vi "ReadDAQTask.vi"(8 "Error In":errorcluster, 11 "DAQ Task In":refnum<k21>) -> (0 "Error Out":errorcluster, 2 "Data":dbl[][](array[numeric]), 3 "DAQ Task Out":refnum<k21>)   [LabVIEW 2012]
uses:
  <vilib>/DAQmx/read.llb/DAQmx Read (Analog 2D DBL NChan NSamp).vi
  <vilib>/DAQmx/miscellaneous.llb/DAQmx Fill In Error Info.vi
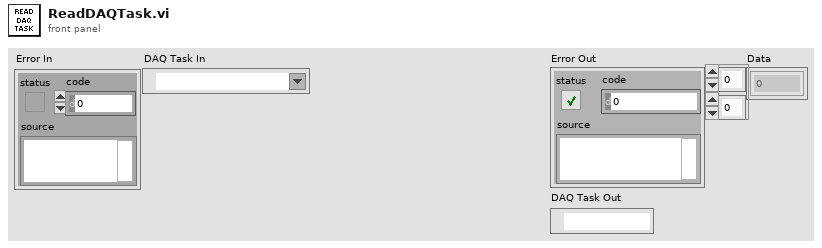
[diagram p1: front panel]
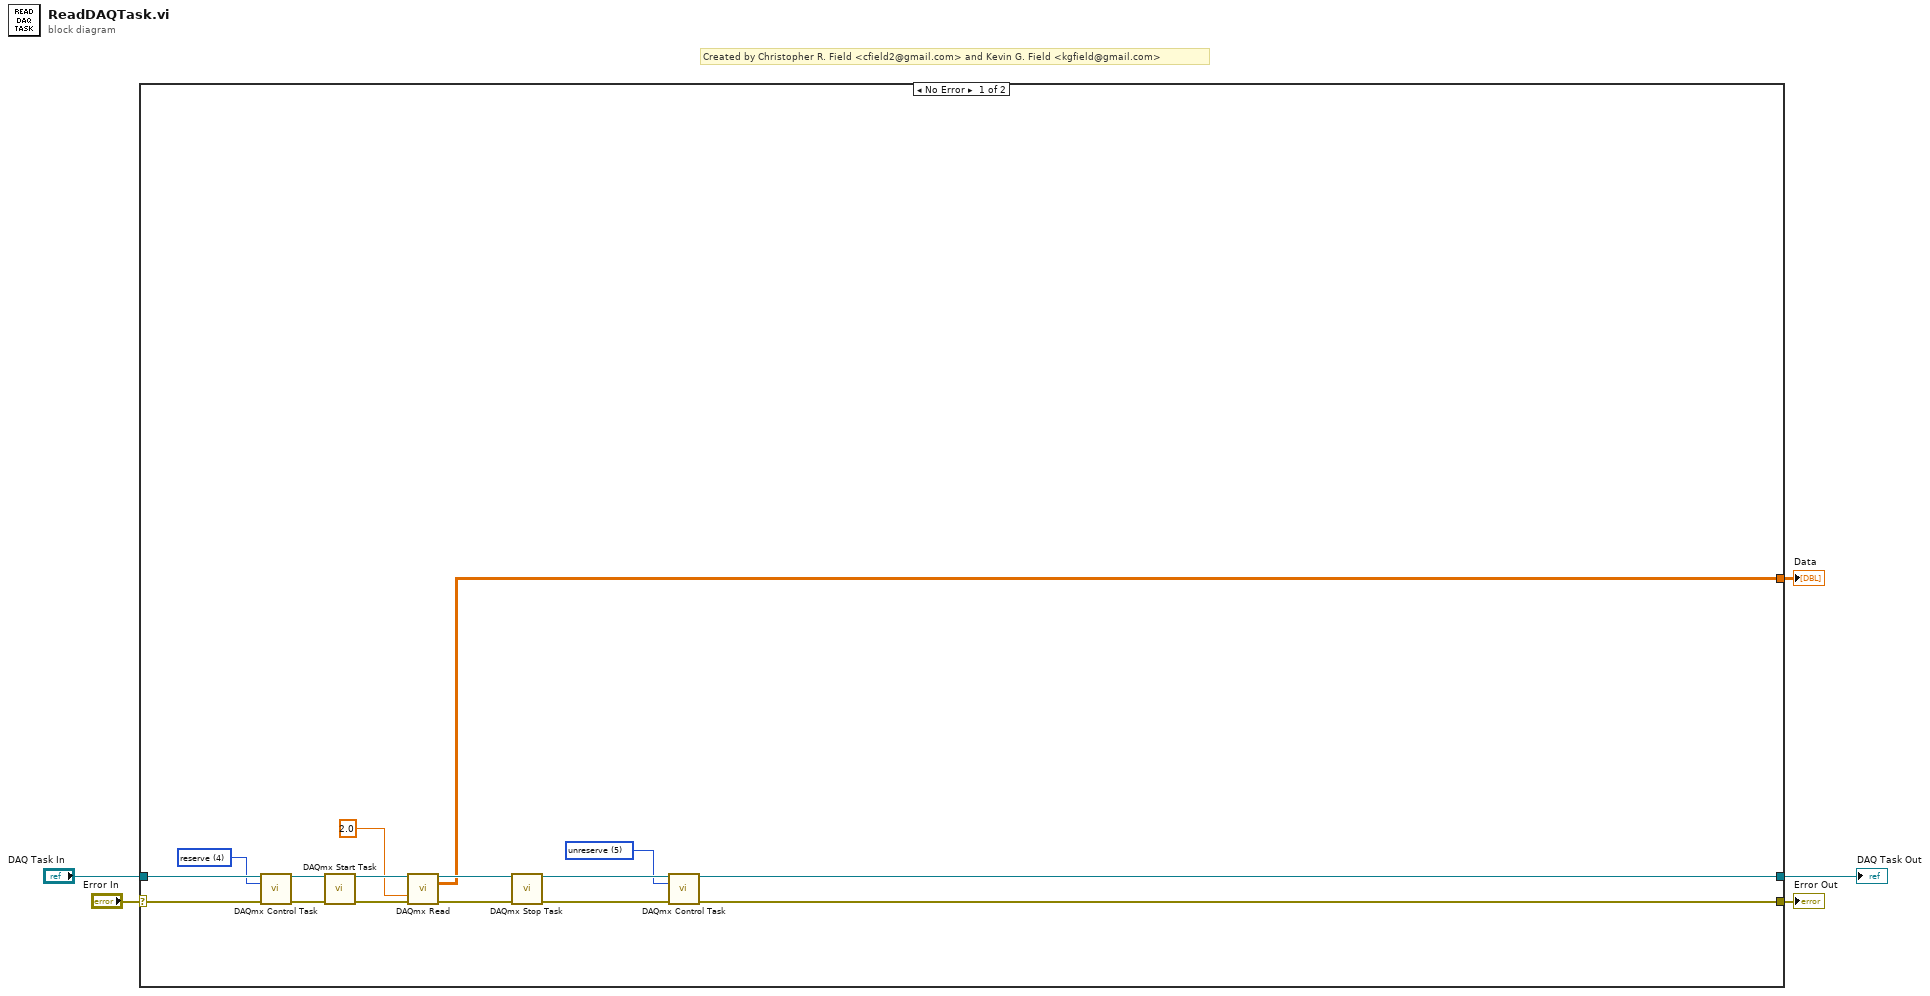
[diagram p0: block diagram]
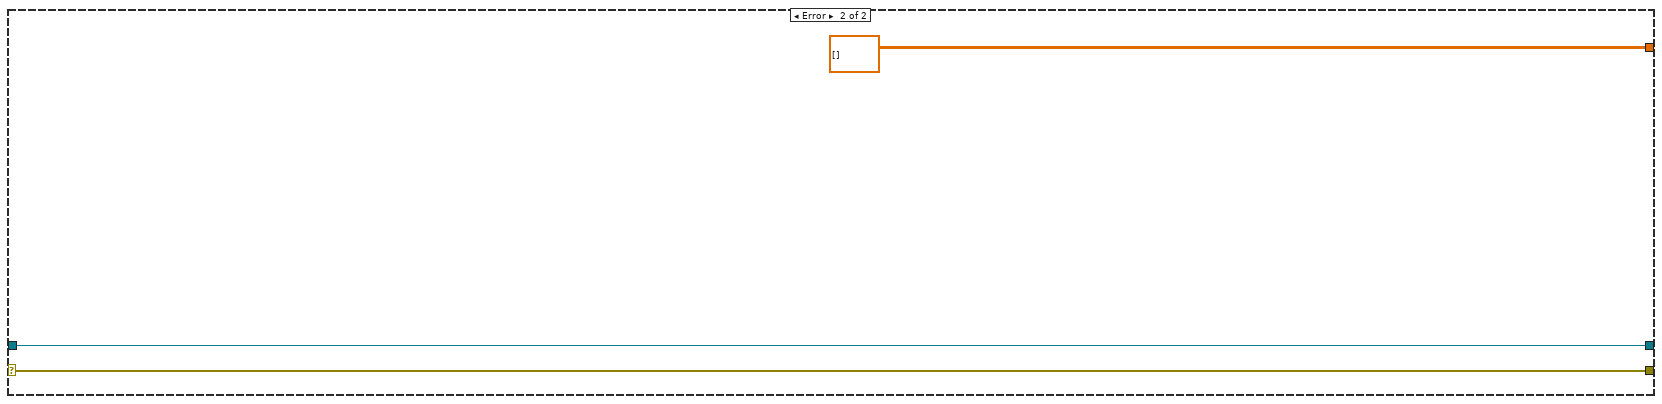
[diagram p2: hidden frame]
diagram:
  # "Created by Christopher R. Field <cfield2@gmail.com> and Kevin G. Field <kgfield@gmail.com>"
  n1 = case shown="No Error" "Error In" {
    selector: "Error In" -> [w11 w23]
    tunnel: [w8 w23] -> w4
    tunnel: "DAQ Task In" -> [w14 w24]
    tunnel: [w7 w24] -> w2
    tunnel: [w17 dbl[][] [] ("data")] -> w1
    frame No Error {
      w9 = 5 items=["verify"=2, "reserve"=4, "commit"=3, "unreserve"=5, "abort"=6] ("action")
      w10 = 4 items=["verify"=2, "reserve"=4, "commit"=3, "unreserve"=5, "abort"=6] ("action")
      n2 = call <vilib>:"DAQmx Control Task.vi"("task/channels in"=w14, "action"=w10, "error in"=w11) -> ("task out"=w13:refnum<k21>, "error out"=w12:errorcluster)  [unwired: 11 in]
      n3 = call <vilib>:"DAQmx Start Task.vi"("task/channels in"=w13, "error in"=w12) -> ("task out"=w21:refnum<k21>, "error out"=w20:errorcluster)  [unwired: 12 in]
      n4 = call-poly <vilib>:"DAQmx Read.vi"("task/channels in"=w21, "timeout"=2.0, "error in"=w20) -> ("task out"=w19:refnum<k21>, "data"=w17:dbl[][], "error out"=w18:errorcluster)  [unwired: 10 in]
      n5 = call <vilib>:"DAQmx Stop Task.vi"("task/channels in"=w19, "error in"=w18) -> ("task out"=w16:refnum<k21>, "error out"=w15:errorcluster)  [unwired: 12 in]
      n6 = call <vilib>:"DAQmx Control Task.vi"("task/channels in"=w16, "action"=w9, "error in"=w15) -> ("task out"=w7:refnum<k21>, "error out"=w8:errorcluster)  [unwired: 11 in]
    }
    frame Error {
    }
  }
  "Error Out" <- w4
  "DAQ Task Out" <- w2
  "Data" <- w1
